vi "Lidar Finder_FINAL.vi"(3 "Stop":bool, 4 "Find Objects":bool, 5 "VISA resource name":refnum<visa-resource-name>="Hukuyo") -> (0 "Objects":cluster{i32, i32}[](array[cluster]), 1 "Widest Object":cluster{i32, i32}, 2 "Where to Point":i32)   [LabVIEW 2014]
uses:
  <instrlib>/Hokuyo URG Series/Public/Initialize-Standard.vi
  <instrlib>/Hokuyo URG Series/Hokuyo URG Series.lvlib
panel:
  in  "threshold":dbl=-180.0
  in  "Tab Control":enum32{"Raw Data", "Clean Data"}(tab)
  out "Data Aquired":picture
  out "Object Graph":i32[](graph)
  out "Edges":i32[](graph)
  out "threshold_val":dbl
  out "Blinky LIDAR  Running":bool
  in  "polar attributes (hidden)":T1={"maximum"=30000.0, "minimum"=0.0, "clip to min"=FALSE, "log?(F)"=TRUE, "grid color"=6710886, "plot color"=65280, "fmt and prec"={"format"=enum."Decimal", "precision"=0}, "visible section"=8} {"minimum" format="%0.2f"; "maximum" format="%0.2f"}
  in  "Grid Color":u32(colorbox)=11776947
  in  "Plot Color":u32(colorbox)=14422272
  in  "Max (m)":dbl=1.0
  in  "End Point":dbl=40.0
  in  "Start Point":dbl=-32.0
  in  "Cluster Count":dbl=1.0
  in  "Encoding Width":u16(ring)=3 items=["2 Byte"=2, "3 Byte"=3]
  # "click here to run"
  # "Hokuyo LIDAR Example"
  # "Plot in mm"
  # "start at-32"
  # "start at 40"
  # "Start with 1.0 m"
  # "Find Gaps"
  # "set to -180"
  # "Hokuyo plugged in?"
  # "Location"
  # "Width"
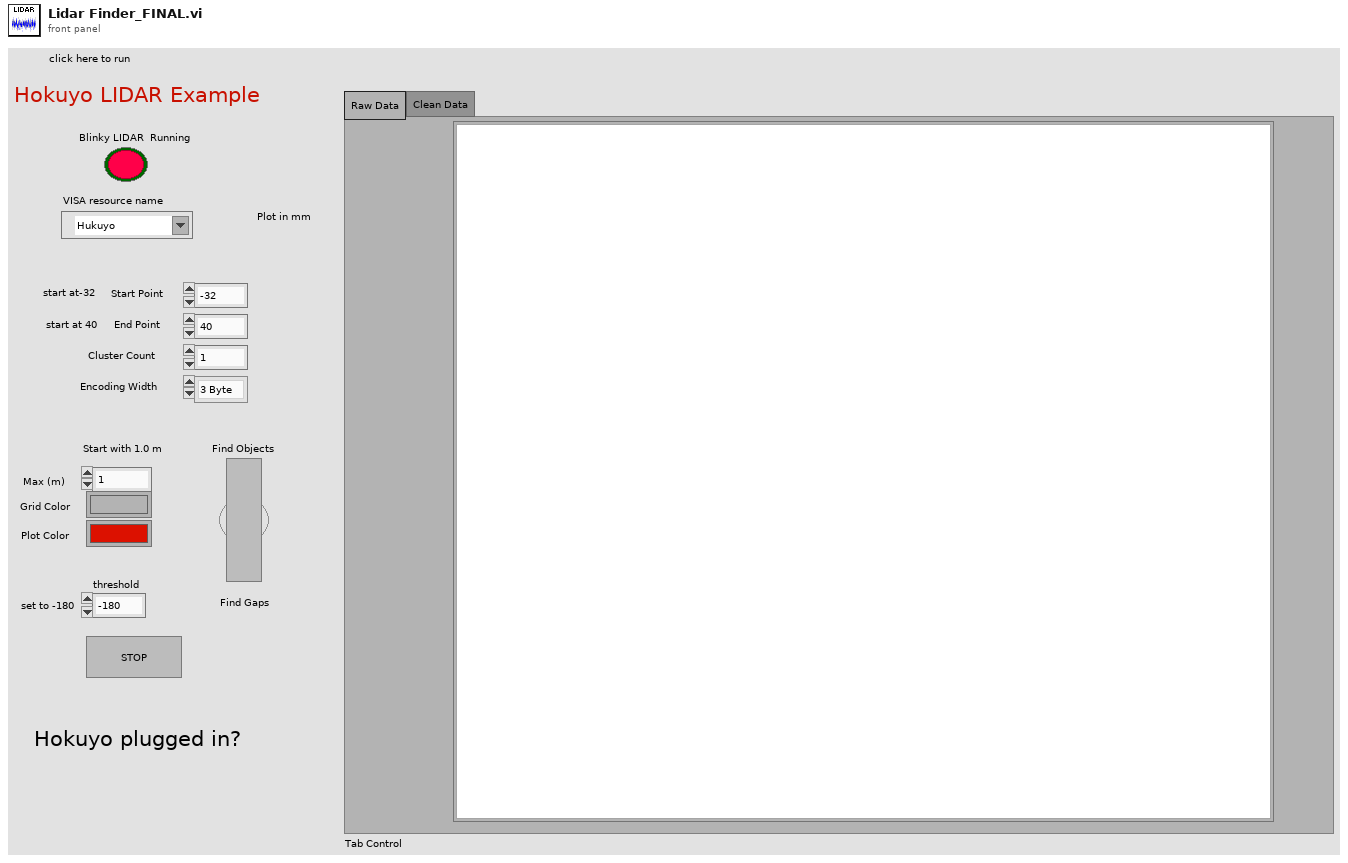
[diagram p1: front panel]
types:
  T1 = cluster{"maximum":dbl, "minimum":dbl, "clip to min":bool, "log?(F)":bool, "grid color":u32, "plot color":u32, "fmt and prec":cluster{"format":enum8{"Decimal", "Scientific", "Engineering", "Binary", "Octal", "Hex"}, "precision":u8}, "visible section":u16}
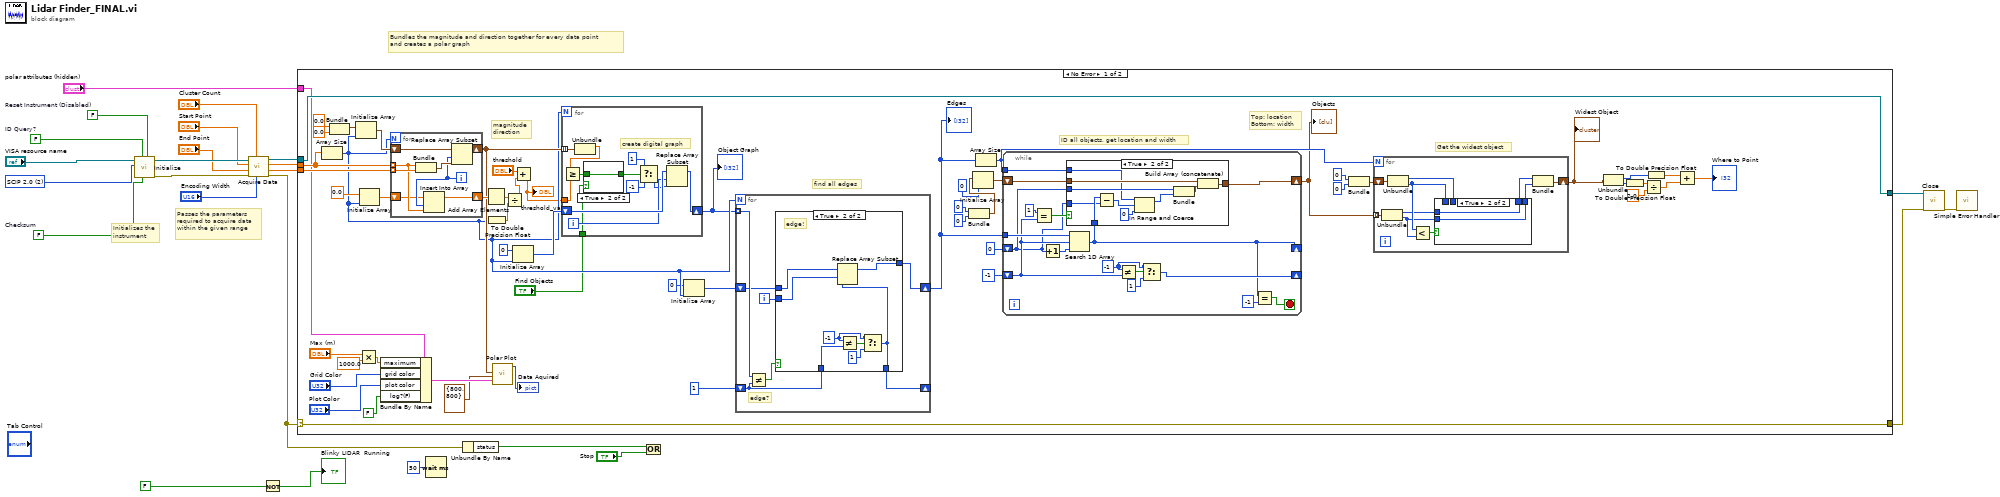
[diagram p0: block diagram]
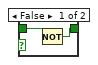
[diagram p5: hidden frame]
diagram:
  w22 = FALSE  # Checksum
  w20 = FALSE  # ID Query?
  w18 = u32 2 items=["Convert to Latest", "SCIP 1.1", "SCIP 2.0"] ("Protocol")
  w19 = FALSE  # Reset Instrument (Disabled)
  # "Passes the parameters\nrequired to acquire data\nwithin the given range"
  # "Bundles the magnitude and direction together for every data point\nand creates a polar graph"
  # "Initializes the instrument"
  n1 = call-poly <instrlib>:"Initialize.vi"("Reset? (F: No)"=w19, "Checksum (Disabled)"=w22, "ID Query? (Enabled)"=w20, "Protocol (2: SCIP 2.0)"=w18, "VISA resource name"="VISA resource name") -> ("error out"=w15:errorcluster, "VISA resource name out"=w16:refnum<visa-resource-name>)  [unwired: 5 in]
  n2 = call <instrlib>:"Acquire Data.vi"("Data Encoding Width (3 Byte)"="Encoding Width", "Cluster Count (1)"="Cluster Count", "error in (no error)"=w15, "End Point (120°)"="End Point", "Start Point (-120°)"="Start Point", "VISA resource name"=w16) -> ("error out"=w7:errorcluster, "Direction"=w8:dbl[], "Magnitude"=w9:dbl[], "VISA resource name out"=w10:refnum<visa-resource-name>)  [unwired: 2 in]
  n3 = Not(x=FALSE) -> (.not. x?=→"Blinky LIDAR  Running":bool)
  n4 = case shown="No Error" w7 {
    selector: w7 -> [w78 w163]
    tunnel: [w78 w163] -> w24
    tunnel: w10 -> [w79 w162]
    tunnel: [w79 w162] -> w17
    tunnel: w9 -> [w73 _]
    tunnel: w8 -> [w72 _]
    tunnel: "polar attributes (hidden)" -> [w70 _]
    frame No Error {
      # "Get the widest object"
      # "Top: location\nBottom: width"
      # "find all edges"
      # "ID all objects, get location and width"
      # "magnitude\ndirection"
      n5 = Array Size(array=w73) -> (size(s)=w53:i32)
      n6 = Bundle(0.0, 0.0) -> (w75:cluster{dbl, dbl})  [unwired: 1 in]
      n7 = Initialize Array(w75, w53) -> (w74:cluster{dbl, dbl}[])
      n8 = Multiply(x="Max (m)", y=1000.0) -> (x*y=w66:dbl)
      n9 = Initialize Array(0.0, w53) -> (w61:dbl[])
      n10 = Bundle By Name(cluster=w70, "maximum"=w66, "grid color"="Grid Color", "plot color"="Plot Color", "log?(F)"=FALSE) -> (w71:T1)
      n11 = for {
        N: w53 -> [_]
        shift-right: [w159] -> w57
        shift-left: w74 -> [w160]
        tunnel: w73 -> [w156] mode=indexing
        tunnel: w72 -> [w161] mode=indexing
        shift-right: [w154] -> w60
        shift-left: w61 -> [w155]
        i -> [w157]
        n12 = Bundle(w156, w161) -> (w158:cluster{dbl, dbl})  [unwired: 1 in]
        n13 = Insert Into Array(array=w155, index=w157, new element=w156) -> (w154:dbl[])
        n14 = Replace Array Subset(array=w160, new element=w158, index=w157) -> (w159:cluster{dbl, dbl}[])
      }
      n15 = Add Array Elements(numeric array=w60) -> (sum=w59:dbl)
      n16 = To Double Precision Float(number=w53) -> (double precision float=w58:dbl)
      n17 = call <vilib>:"Polar Plot.vi"("polar attributes"=w71, "dimensions (w,h)"=cluster{"width":i16, "height":i16} {"width"=800, "height"=800}, "data array [mag, phase (deg)]"=w57) -> ("new picture"=→"Data Aquired":picture)  [unwired: 8 in]
      n18 = Divide(x=w59, y=w58) -> (x/y=w26:dbl)
      n19 = Initialize Array(0, w53) -> (w56:i32[])
      n20 = Add(x="threshold", y=w26) -> (x+y=w27:dbl)
      "threshold_val" <- w27
      n21 = for {
        N: w53 -> [_]
        tunnel: w57 -> [w150] mode=indexing
        tunnel: w27 -> [w148]
        shift-right: [w145] -> w50
        shift-left: w56 -> [w147]
        tunnel: "Find Objects" -> [w139]
        i -> [w146]
        # "create digital graph"
        n22 = Unbundle(w150) -> (w149:dbl)  [unwired: 1 out]
        n23 = Greater Or Equal?(x=w149, y=w148) -> (x >= y?=w141:bool)
        n24 = case shown="True" w139 {
          tunnel: w141 -> [w152 w153]
          tunnel: [w151 w153] -> w140
          frame False {
            n25 = Not(x=w152) -> (.not. x?=w151:bool)
          }
          frame True {
          }
        }
        n26 = Select(t=1, s=w140, f=-1) -> (s? t:f=w144:i32)
        n27 = Replace Array Subset(array=w147, new element=w144, index=w146) -> (w145:i32[])
      }
      "Object Graph" <- w50
      n28 = Initialize Array(0, w53) -> (w51:i32[])
      n29 = for {
        N: w53 -> [_]
        shift-right: [w126] -> _
        shift-left: 1 -> [w125]
        tunnel: w50 -> [w127] mode=indexing
        shift-right: [w122] -> w42
        shift-left: w51 -> [w124]
        i -> [w123]
        # "edge?"
        n30 = Not Equal?(x=w127, y=w125) -> (x != y?=w128:bool)
        n31 = case shown="True" w128 {
          tunnel: [w130 w132] -> w126
          tunnel: w125 -> [w130 w138]
          tunnel: w124 -> [w129 w134]
          tunnel: w123 -> [_ w133]
          tunnel: [w129 w131] -> w122
          frame False {
            # "no edge"
          }
          frame True {
            w136 = -1
            # "edge!"
            n32 = Not Equal?(x=w136, y=w138) -> (x != y?=w137:bool)
            n33 = Select(t=w136, s=w137, f=1) -> (s? t:f=w132:i32)
            n34 = Replace Array Subset(array=w134, new element=w132, index=w133) -> (w131:i32[])
          }
        }
      }
      "Edges" <- w42
      n35 = Bundle(0, 0) -> (w46:cluster{i32, i32})  [unwired: 1 in]
      n36 = Initialize Array(w46, 0) -> (w47:cluster{i32, i32}[])
      n37 = Array Size(array=w42) -> (size(s)=w41:i32)
      n38 = while {
        tunnel: w42 -> [w108]
        shift-right: [w104] -> _
        shift-left: -1 -> [w99]
        shift-right: [w101] -> _
        shift-left: 0 -> [w96]
        shift-right: [w103] -> w37
        shift-left: w47 -> [w102]
        tunnel: w41 -> [w95]
        stop <- w110 stop-if-true
        w106 = -1
        n39 = Equal?(x=1, y=w99) -> (x = y?=w98:bool)
        n40 = Increment(x=w96) -> (x+1=w97:i32)
        n41 = Search 1D Array(1D array=w108, element=w99, start index (0)=w97) -> (index of element=w101:i32)
        n42 = case shown="True" w98 {
          tunnel: [w111 w121] -> w103
          tunnel: w102 -> [w111 w120]
          tunnel: w101 -> [_ w118]
          tunnel: w96 -> [_ w117]
          tunnel: w96 -> [_ w116]
          tunnel: w95 -> [_ w115]
          frame False {
          }
          frame True {
            n43 = Subtract(x=w118, y=w117) -> (x-y=w114:i32)
            n44 = In Range and Coerce(upper limit=w115, x=w114, lower limit=0) -> (coerced(x)=w113:i32)  [unwired: 1 out]
            n45 = Bundle(w116, w113) -> (w119:cluster{i32, i32})  [unwired: 1 in]
            n46 = Build Array (concatenate)(w120, w119) -> (w121:cluster{i32, i32}[])
          }
        }
        n47 = Not Equal?(x=w106, y=w99) -> (x != y?=w105:bool)
        n48 = Select(t=w106, s=w105, f=1) -> (s? t:f=w104:i32)
        n49 = Equal?(x=w101, y=-1) -> (x = y?=w110:bool)
      }
      "Objects" <- w37
      n50 = Bundle(0, 0) -> (w38:cluster{i32, i32})  [unwired: 1 in]
      n51 = for {
        N: w41 -> [_]
        shift-right: [w89] -> w36
        shift-left: w38 -> [w90]
        tunnel: w37 -> [w85] mode=indexing
        n52 = Unbundle(w85) -> (w82:i32, w81:i32)
        n53 = Unbundle(w90) -> (w87:i32, w83:i32)
        n54 = Less?(x=w83, y=w81) -> (x < y?=w84:bool)
        n55 = case shown="True" w84 {
          tunnel: [w92 w94] -> w88
          tunnel: w87 -> [w92 _]
          tunnel: [w91 w93] -> w86
          tunnel: w83 -> [w91 _]
          tunnel: w82 -> [_ w94]
          tunnel: w81 -> [_ w93]
          frame False {
          }
          frame True {
          }
        }
        n56 = Bundle(w88, w86) -> (w89:cluster{i32, i32})  [unwired: 1 in]
      }
      "Widest Object" <- w36
      n57 = Unbundle(w36) -> (w30:i32, w34:i32)
      n58 = To Double Precision Float(number=w34) -> (double precision float=w33:dbl)
      n59 = Divide(x=w33, y=2.0) -> (x/y=w31:dbl)
      n60 = To Double Precision Float(number=w30) -> (double precision float=w29:dbl)
      n61 = Add(x=w29, y=w31) -> (x+y=→"Where to Point":dbl)
    }
    frame Error {
    }
  }
  n62 = Wait (ms)(milliseconds to wait=u32 50) -> ()  [unwired: 1 out]
  n63 = Unbundle By Name(w7) -> ("status"=w12:bool)
  n64 = Or(x=w12, y="Stop") -> ()  [unwired: 1 out]
  n65 = call <instrlib>:"Close.vi"("error in (no error)"=w24, "VISA resource name"=w17) -> ("error out"=w21:errorcluster)  [unwired: 9 in]
  n66 = call <vilib>:"Simple Error Handler.vi"("error in (no error)"=w21) -> ()  [unwired: 4 in, 5 out]
